vi "add_attribute_name_to_error_message.vi"(7 "Attribute":T1={"Identifier"="", "Descriptive name"="", "Data Type"=enum."Integer 32", "Command"="", "Access"=2, "Range Table"="", "Read Callback"="", "Write Callback"="", "Range Callback"="", "Check Callback"="", "Rngtable Callback"="", "Coerce Callback"="", "Supported Models"="", "Instrument Options"="", "Repeated Capabilities"="", "Check Status Callback"="", "Index"=0, "Flag: OPC Wait"=FALSE, "Flag: Dont check status"=FALSE, "Flag: Cache Only"=FALSE} {"Access" items=["Read Only", "Write Only", "Read/Write"]}, 8 "error in":errorcluster, 11 "Recompose even if original message\nalready contains an attribute name (F)":bool) -> (0 "error out":errorcluster, 3 "Recomposed":bool)   [LabVIEW 2014, in "rszvl_rsidr_core.lvlib"]
uses:
  rszvl_rsidr_core.lvlib
  type_Attribute.ctl
  type_Attribute_Data_Type.ctl
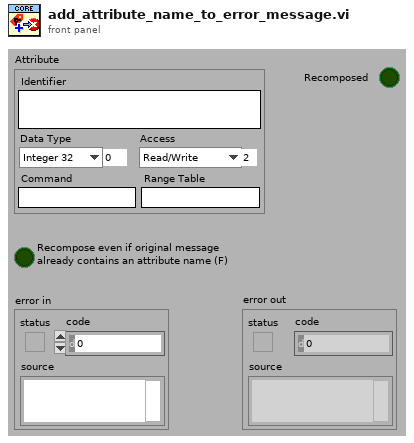
[diagram p1: front panel]
types:
  T1 = typedef "rszvl_rsidr_core.lvlib/type_Attribute.ctl" = cluster{"Identifier":string, "Descriptive name":string, "Data Type":T2, "Command":string, "Access":u16, "Range Table":string, "Read Callback":string, "Write Callback":string, "Range Callback":string, "Check Callback":string, "Rngtable Callback":string, "Coerce Callback":string, "Supported Models":string, "Instrument Options":string, "Repeated Capabilities":string, "Check Status Callback":string, "Index":i32, "Flag: OPC Wait":bool, "Flag: Dont check status":bool, "Flag: Cache Only":bool}
  T2 = typedef "rszvl_rsidr_core.lvlib/type_Attribute_Data_Type.ctl" = enum16{"Integer 32", "Double", "String", "Boolean", "None", "Integer 64"}
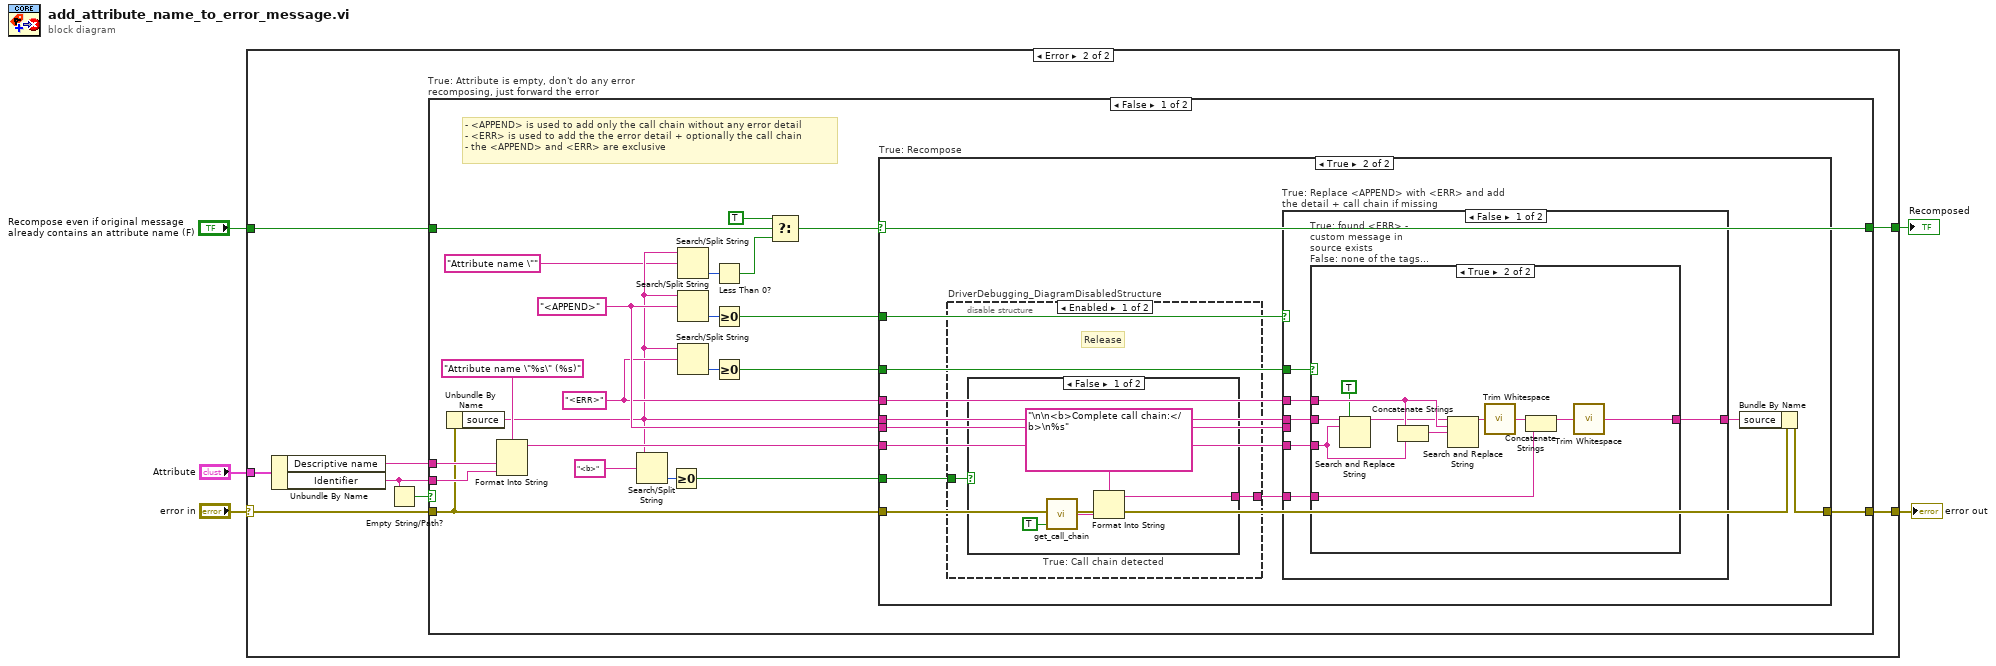
[diagram p0: block diagram]
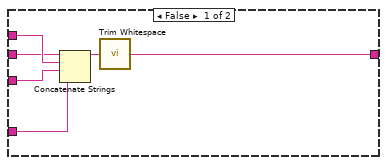
[diagram p6: hidden frame]
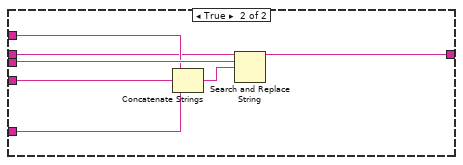
[diagram p7: hidden frame]
diagram:
  n1 = case shown="Error" "error in" {
    selector: "error in" -> [w6 w12]
    tunnel: [w6 w14] -> w5
    tunnel: "Attribute" -> [_ w9]
    tunnel: "Recompose even if original message\nalready contains an attribute name (F)" -> [_ w8]
    tunnel: [_ w7] -> w1
    frame No Error {
    }
    frame Error {
      n2 = Unbundle By Name(w9) -> ("Descriptive name"=w13:string, "Identifier"=w10:string)
      n3 = Empty String/Path?(string/path=w10) -> (empty?=w11:bool)
      n4 = case "True: Attribute is empty, don't do any error recomposing, just forward the error" shown="False" w11 {
        tunnel: [w23 w85] -> w14
        tunnel: w10 -> [w32 _]
        tunnel: w13 -> [w30 _]
        tunnel: w12 -> [w24 w85]
        tunnel: w8 -> [w18 _]
        tunnel: [w15 _] -> w7
        frame False {
          w28 = "<ERR>" ("search string/char (-)")
          w29 = "<APPEND>" ("search string/char (-)")
          # "- <APPEND> is used to add only the call chain without any error detail\n- <ERR> is used to add the the error detail + optionally the call chain\n- the <APPEND> and <ERR> are exclusive"
          n5 = Unbundle By Name(w24) -> ("source"=w21:string)
          n6 = Format Into String(format string="Attribute name \"%s\" (%s)", w30, w32) -> (resulting string=w27:string)  [unwired: 2 in, 1 out]
          n7 = Search/Split String(string=w21, search string/char (-)="<b>" ("call chain beginning string")) -> (offset of match=w26:i32)  [unwired: 1 in, 2 out]
          n8 = Greater Or Equal To 0?(x=w26) -> (x >= 0?=w22:bool)
          n9 = Search/Split String(string=w21, search string/char (-)="Attribute name \"") -> (offset of match=w19:i32)  [unwired: 1 in, 2 out]
          n10 = Search/Split String(string=w21, search string/char (-)=w29) -> (offset of match=w36:i32)  [unwired: 1 in, 2 out]
          n11 = Search/Split String(string=w21, search string/char (-)=w28) -> (offset of match=w34:i32)  [unwired: 1 in, 2 out]
          n12 = Less Than 0?(x=w19) -> (x < 0?=w16:bool)
          n13 = Greater Or Equal To 0?(x=w36) -> (x >= 0?=w35:bool)
          n14 = Greater Or Equal To 0?(x=w34) -> (x >= 0?=w33:bool)
          n15 = Select(t=TRUE ("f"), s=w18, f=w16) -> (s? t:f=w15:bool)
          n16 = case "True: Recompose" shown="True" w15 {
            tunnel: w35 -> [_ w48]
            tunnel: w33 -> [_ w47]
            tunnel: w29 -> [_ w46]
            tunnel: w28 -> [_ w45]
            tunnel: w27 -> [_ w44]
            tunnel: w24 -> [w37 w42]
            tunnel: [w37 w41] -> w23
            tunnel: w22 -> [_ w40]
            tunnel: w21 -> [_ w38]
            frame False {
            }
            frame True {
              n17 = disable-structure "DriverDebugging_DiagramDisabledStructure" shown="Enabled" {
                disable-tunnel: w40 -> [w50 _]
                disable-tunnel: [w49 _] -> w39
                frame Enabled {
                  # "Release"
                  n18 = case "True: Call chain detected" shown="False" w50 {
                    tunnel: [w51 _] -> w49
                    frame False {
                      n19 = call "get_call_chain.vi"("Remove lvlib names (F)"=TRUE) -> ("Call chain out in spreadsheet string"=w53:string)  [unwired: 2 in, 2 out]
                      n20 = Format Into String(format string="\n\n<b>Complete call chain:</b>\n%s", w53) -> (resulting string=w51:string)  [unwired: 2 in, 1 out]
                    }
                    frame True {
                    }
                  }
                }
                frame Disabled {
                  # "Debug"
                }
              }
              n21 = case "True: Replace <APPEND> with <ERR> and add the detail + call chain if missing" shown="False" w48 {
                tunnel: w47 -> [w60 _]
                tunnel: w38 -> [w59 w80]
                tunnel: w46 -> [_ w84]
                tunnel: w45 -> [w58 w83]
                tunnel: w44 -> [w57 w82]
                tunnel: [w56 w81] -> w43
                tunnel: w39 -> [w55 w78]
                frame False {
                  n22 = case "True: found <ERR> - custom message in source exists\nFalse: none of the tags found, compose the message completely new" shown="True" w60 {
                    tunnel: w59 -> [w63 w75]
                    tunnel: w58 -> [w65 w77]
                    tunnel: w57 -> [w64 w73]
                    tunnel: [w66 w76] -> w56
                    tunnel: w55 -> [w61 w71]
                    frame False {
                      n23 = Concatenate Strings(w63, w65, w64, w61) -> (w62:string)
                      n24 = call "Trim Whitespace.vi"("string"=w62) -> ("trimmed string"=w66:string)  [unwired: 1 in]
                    }
                    frame True {
                      n25 = Search and Replace String(replace all?=TRUE ("replace all? (F)"), input string=w75, search string=w73) -> (result string=w72:string)  [unwired: 5 in, 3 out]
                      n26 = Concatenate Strings(w77, w73) -> (w69:string)
                      n27 = Search and Replace String(input string=w72, search string=w77, replace string=w69) -> (result string=w70:string)  [unwired: 5 in, 3 out]
                      n28 = call "Trim Whitespace.vi"("string"=w70) -> ("trimmed string"=w68:string)  [unwired: 1 in]
                      n29 = Concatenate Strings(w68, w71) -> (w67:string)
                      n30 = call "Trim Whitespace.vi"("string"=w67) -> ("trimmed string"=w76:string)  [unwired: 1 in]
                    }
                  }
                }
                frame True {
                  n31 = Concatenate Strings(w83, w82, w78) -> (w79:string)
                  n32 = Search and Replace String(input string=w80, search string=w84, replace string=w79) -> (result string=w81:string)  [unwired: 5 in, 3 out]
                }
              }
              n33 = Bundle By Name(cluster=w42, "source"=w43) -> (w41:errorcluster)
            }
          }
        }
        frame True {
        }
      }
    }
  }
  "error out" <- w5
  "Recomposed" <- w1
